vi "tokenizer.vi"(1 "Input String":string) -> (0 "Output Array":string[](array[string]))   [LabVIEW 2010]
uses:
  <vilib>/Utility/error.llb/whitespace.ctl
panel:
  out "Token":string
  out "Output":string
  # "1) LINE<space>[Displacement]<space>[Speed]<space>[Current]"
  # "2) JUMP<space>[Displacement]<space>[Speed]"
  # "3) ARC<space>[Type]<space>[Radius]<space>[Current]"
  # "4) LINE1<space>[Displacement]<space>[Speed]<space>[Current]<space>[t_before]<space>[t_enable]<space>[Frequency]<space>[DTY]<space>[HIL]<space>[LOL]"
  # "5) LINE2<space>[Displacement]<space>[Speed]<space>[Current]<space>[t_before]<space>[frequency]<space>[Amplitude]<space>[t_enable]"
  # "6) WAIT<space>[Time]"
  # "1"
  # "2"
  # "3"
  # "4"
  # "5"
  # "6"
  # "7"
  # "8"
  # "9"
  # "10"
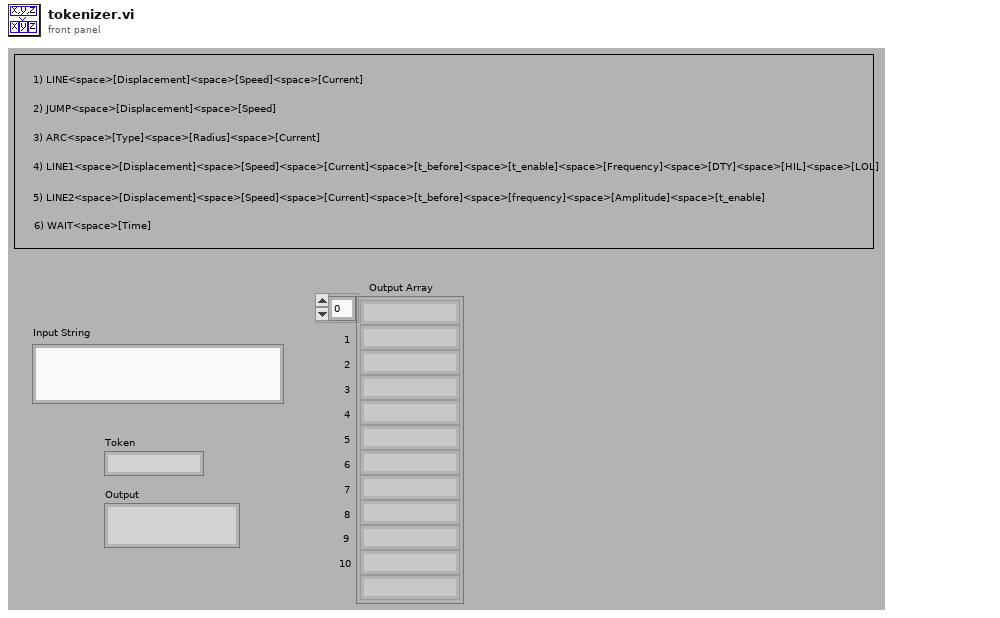
[diagram p1: front panel]
types:
  T1 = typedef "whitespace.ctl" = u16
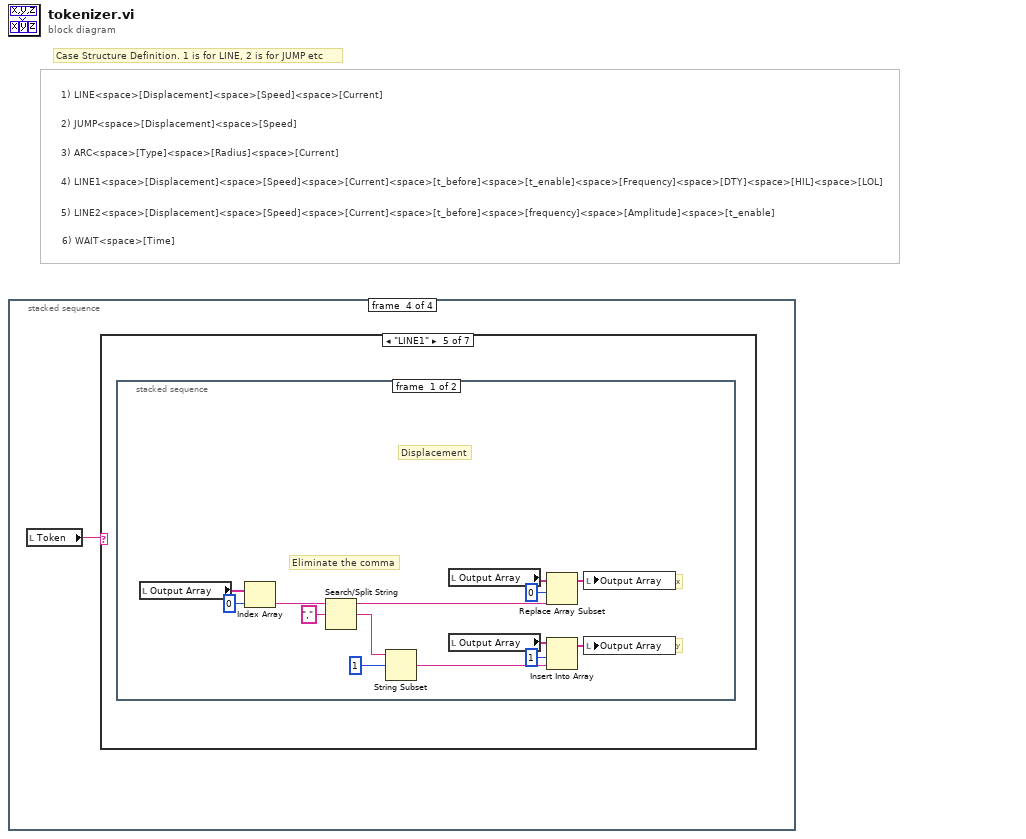
[diagram p0: block diagram]
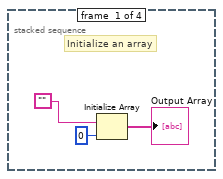
[diagram p2: hidden frame]
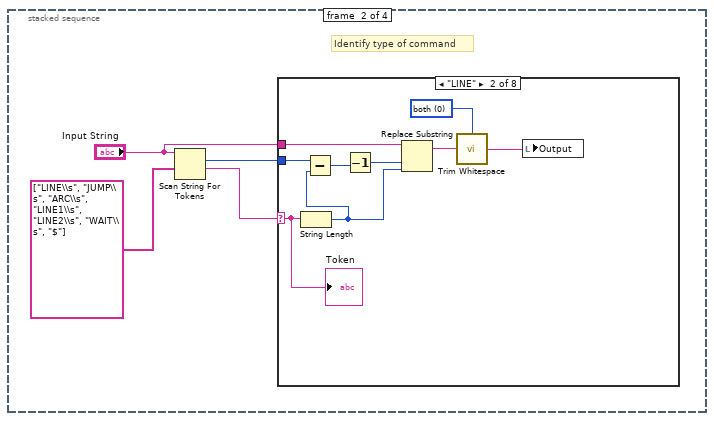
[diagram p3: hidden frame]
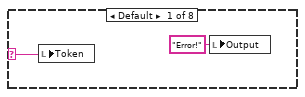
[diagram p4: hidden frame]
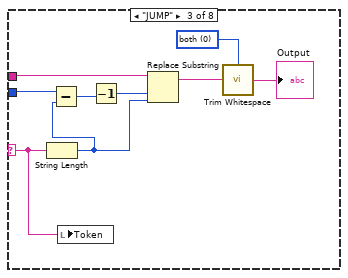
[diagram p5: hidden frame]
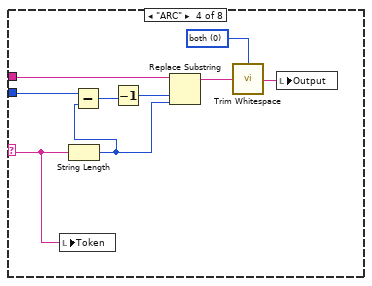
[diagram p6: hidden frame]
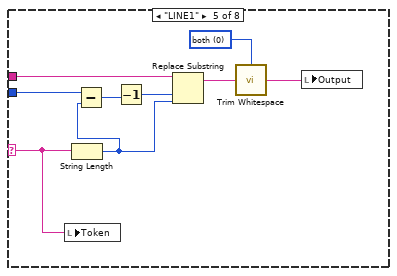
[diagram p7: hidden frame]
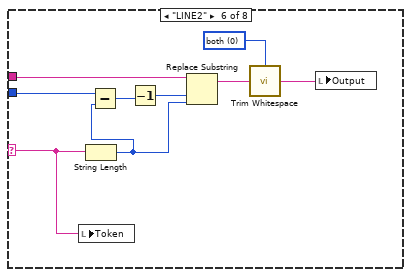
[diagram p8: hidden frame]
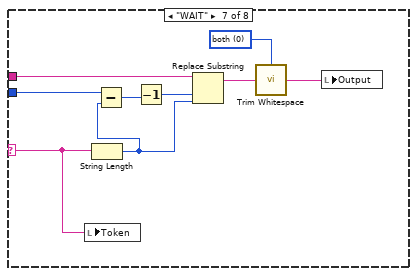
[diagram p9: hidden frame]
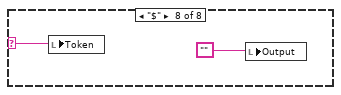
[diagram p10: hidden frame]
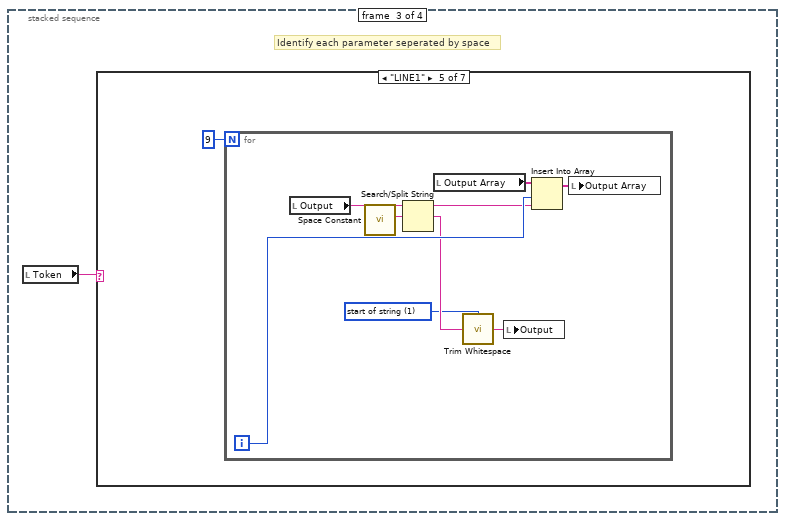
[diagram p11: hidden frame]
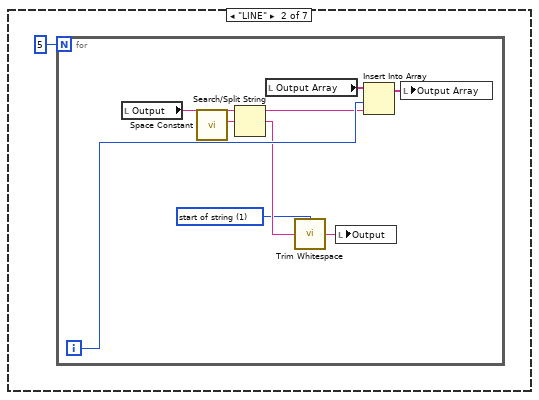
[diagram p13: hidden frame]
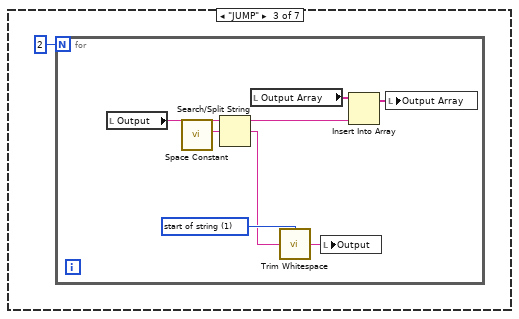
[diagram p14: hidden frame]
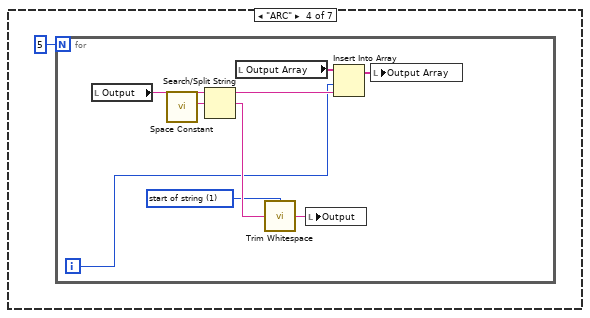
[diagram p15: hidden frame]
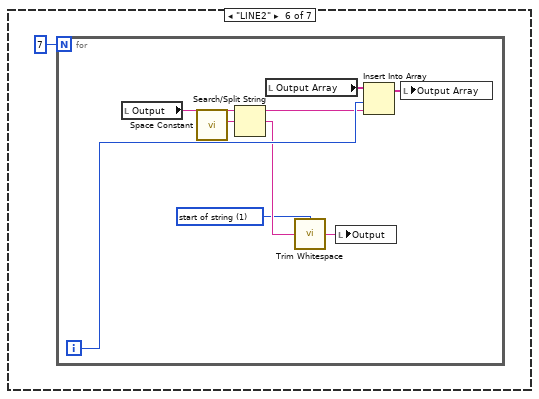
[diagram p16: hidden frame]
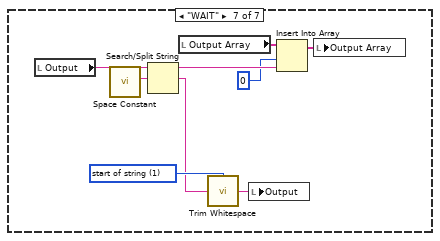
[diagram p17: hidden frame]
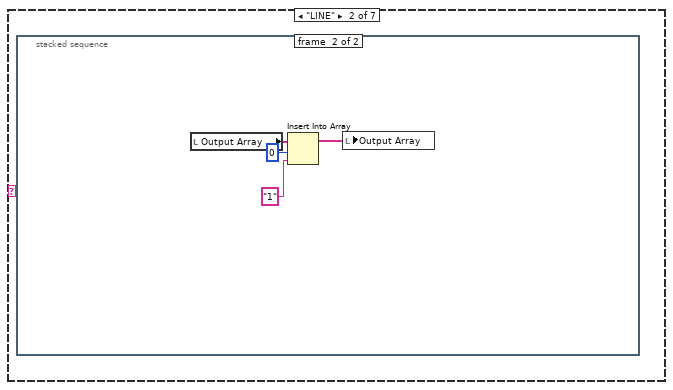
[diagram p19: hidden frame]
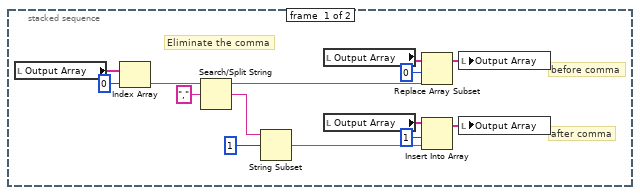
[diagram p20: hidden frame]
diagram:
  # "Case Structure Definition. 1 is for LINE, 2 is for JUMP etc"
  # "6) WAIT<space>[Time]"
  # "5) LINE2<space>[Displacement]<space>[Speed]<space>[Current]<space>[t_before]<space>[frequency]<space>[Amplitude]<space>[t_enable]"
  # "4) LINE1<space>[Displacement]<space>[Speed]<space>[Current]<space>[t_before]<space>[t_enable]<space>[Frequency]<space>[DTY]<space>[HIL]<space>[LOL]"
  # "3) ARC<space>[Type]<space>[Radius]<space>[Current]"
  # "2) JUMP<space>[Displacement]<space>[Speed]"
  # "1) LINE<space>[Displacement]<space>[Speed]<space>[Current]"
  n1 = stacked-sequence {
    frame #0 {
      # "Initialize an array"
      n2 = Initialize Array("", 0 ("dimension size")) -> (→"Output Array":string[])
    }
    frame #1 {
      # "Identify type of command"
      n3 = Scan String For Tokens(7:string[] ["LINE\\s", "JUMP\\s", "ARC\\s", "LINE1\\s", "LINE2\\s", "WAIT\\s", "$"] ("operators (none)"), 9:"Input String") -> (1:w7:string, 2:w5:i32)  [unwired: 4 in, 2 out]
      n4 = case shown="\"LINE\"" w7 {
        selector: w7 -> [w8 w13 w22 w31 w40 w47 w55 w65]
        tunnel: "Input String" -> [_ w18 w24 w33 w42 w49 w57 _]
        tunnel: w5 -> [_ w17 w23 w32 w41 w48 w56 _]
        frame Default {
          n5 = local write "Token"(w8) -> ()
          n6 = local write "Output"("Error!" ("String")) -> ()
        }
        frame "LINE" {
          w10 = T1 0 items=["both", "start of string", "end of string"] ("location (both)")
          n7 = String Length(string=w13) -> (length=w16:i32)
          n8 = Subtract(x=w17, y=w16) -> (x-y=w15:i32)
          n9 = Decrement(x=w15) -> (x-1=w14:i32)
          n10 = Replace Substring(2:w16, 3:w14, 5:w18) -> (1:w12:string)  [unwired: 1 in, 1 out]
          n11 = call <vilib>:"Trim Whitespace.vi"("string"=w12, "location (both)"=w10) -> ("trimmed string"=w11:string)
          n12 = local write "Output"(w11) -> ()
          "Token" <- w13
        }
        frame "JUMP" {
          w21 = T1 0 items=["both", "start of string", "end of string"] ("location (both)")
          n13 = String Length(string=w22) -> (length=w27:i32)
          n14 = Subtract(x=w23, y=w27) -> (x-y=w26:i32)
          n15 = local write "Token"(w22) -> ()
          n16 = Decrement(x=w26) -> (x-1=w25:i32)
          n17 = Replace Substring(2:w27, 3:w25, 5:w24) -> (1:w20:string)  [unwired: 1 in, 1 out]
          n18 = call <vilib>:"Trim Whitespace.vi"("string"=w20, "location (both)"=w21) -> ("trimmed string"=→"Output":string)
        }
        frame "ARC" {
          w30 = T1 0 items=["both", "start of string", "end of string"] ("location (both)")
          n19 = local write "Token"(w31) -> ()
          n20 = String Length(string=w31) -> (length=w36:i32)
          n21 = Subtract(x=w32, y=w36) -> (x-y=w35:i32)
          n22 = Decrement(x=w35) -> (x-1=w34:i32)
          n23 = Replace Substring(2:w36, 3:w34, 5:w33) -> (1:w28:string)  [unwired: 1 in, 1 out]
          n24 = call <vilib>:"Trim Whitespace.vi"("string"=w28, "location (both)"=w30) -> ("trimmed string"=w29:string)
          n25 = local write "Output"(w29) -> ()
        }
        frame "LINE1" {
          w38 = T1 0 items=["both", "start of string", "end of string"] ("location (both)")
          n26 = local write "Token"(w40) -> ()
          n27 = String Length(string=w40) -> (length=w45:i32)
          n28 = Subtract(x=w41, y=w45) -> (x-y=w44:i32)
          n29 = Decrement(x=w44) -> (x-1=w43:i32)
          n30 = Replace Substring(2:w45, 3:w43, 5:w42) -> (1:w37:string)  [unwired: 1 in, 1 out]
          n31 = call <vilib>:"Trim Whitespace.vi"("string"=w37, "location (both)"=w38) -> ("trimmed string"=w39:string)
          n32 = local write "Output"(w39) -> ()
        }
        frame "LINE2" {
          w46 = T1 0 items=["both", "start of string", "end of string"] ("location (both)")
          n33 = local write "Token"(w47) -> ()
          n34 = String Length(string=w47) -> (length=w54:i32)
          n35 = Subtract(x=w48, y=w54) -> (x-y=w53:i32)
          n36 = Decrement(x=w53) -> (x-1=w52:i32)
          n37 = Replace Substring(2:w54, 3:w52, 5:w49) -> (1:w50:string)  [unwired: 1 in, 1 out]
          n38 = call <vilib>:"Trim Whitespace.vi"("string"=w50, "location (both)"=w46) -> ("trimmed string"=w51:string)
          n39 = local write "Output"(w51) -> ()
        }
        frame "WAIT" {
          w58 = T1 0 items=["both", "start of string", "end of string"] ("location (both)")
          n40 = local write "Token"(w55) -> ()
          n41 = String Length(string=w55) -> (length=w63:i32)
          n42 = Subtract(x=w56, y=w63) -> (x-y=w62:i32)
          n43 = Decrement(x=w62) -> (x-1=w61:i32)
          n44 = Replace Substring(2:w63, 3:w61, 5:w57) -> (1:w59:string)  [unwired: 1 in, 1 out]
          n45 = call <vilib>:"Trim Whitespace.vi"("string"=w59, "location (both)"=w58) -> ("trimmed string"=w60:string)
          n46 = local write "Output"(w60) -> ()
        }
        frame "$" {
          n47 = local write "Token"(w65) -> ()
          n48 = local write "Output"("") -> ()
        }
      }
    }
    frame #2 {
      # "Identify each parameter seperated by space"
      n49 = local read "Token"() -> (w66:string)
      n50 = case shown="\"LINE1\"" w66 {
        frame Default {
        }
        frame "LINE" {
          n51 = for {
            N: 5 -> [_]
            i -> [w74]
            w68 = T1 1 items=["both", "start of string", "end of string"] ("location (both)")
            n52 = local read "Output"() -> (w73:string)
            n53 = call <vilib>:"Space Constant.vi"() -> ("String"=w72:string)
            n54 = Search/Split String(string=w73, search string/char (-)=w72) -> (substring before match=w71:string, match + rest of string=w70:string)  [unwired: 1 in, 1 out]
            n55 = local read "Output Array"() -> (w76:string[])
            n56 = call <vilib>:"Trim Whitespace.vi"("string"=w70, "location (both)"=w68) -> ("trimmed string"=w69:string)
            n57 = local write "Output"(w69) -> ()
            n58 = Insert Into Array(array=w76, index=w74, new element=w71) -> (w75:string[])
            n59 = local write "Output Array"(w75) -> ()
          }
        }
        frame "JUMP" {
          n60 = for {
            N: 2 -> [_]
            w85 = T1 1 items=["both", "start of string", "end of string"] ("location (both)")
            n61 = local read "Output"() -> (w80:string)
            n62 = call <vilib>:"Space Constant.vi"() -> ("String"=w81:string)
            n63 = Search/Split String(string=w80, search string/char (-)=w81) -> (substring before match=w82:string, match + rest of string=w83:string)  [unwired: 1 in, 1 out]
            n64 = local read "Output Array"() -> (w78:string[])
            n65 = call <vilib>:"Trim Whitespace.vi"("string"=w83, "location (both)"=w85) -> ("trimmed string"=w84:string)
            n66 = local write "Output"(w84) -> ()
            n67 = Insert Into Array(array=w78, new element=w82) -> (w79:string[])  [unwired: 1 in]
            n68 = local write "Output Array"(w79) -> ()
          }
        }
        frame "ARC" {
          n69 = for {
            N: 5 -> [_]
            i -> [w87]
            w88 = T1 1 items=["both", "start of string", "end of string"] ("location (both)")
            n70 = local read "Output"() -> (w93:string)
            n71 = call <vilib>:"Space Constant.vi"() -> ("String"=w92:string)
            n72 = Search/Split String(string=w93, search string/char (-)=w92) -> (substring before match=w91:string, match + rest of string=w90:string)  [unwired: 1 in, 1 out]
            n73 = local read "Output Array"() -> (w95:string[])
            n74 = call <vilib>:"Trim Whitespace.vi"("string"=w90, "location (both)"=w88) -> ("trimmed string"=w89:string)
            n75 = local write "Output"(w89) -> ()
            n76 = Insert Into Array(array=w95, index=w87, new element=w91) -> (w94:string[])
            n77 = local write "Output Array"(w94) -> ()
          }
        }
        frame "LINE1" {
          n78 = for {
            N: 9 -> [_]
            i -> [w103]
            w97 = T1 1 items=["both", "start of string", "end of string"] ("location (both)")
            n79 = local read "Output"() -> (w102:string)
            n80 = call <vilib>:"Space Constant.vi"() -> ("String"=w101:string)
            n81 = Search/Split String(string=w102, search string/char (-)=w101) -> (substring before match=w100:string, match + rest of string=w99:string)  [unwired: 1 in, 1 out]
            n82 = local read "Output Array"() -> (w105:string[])
            n83 = call <vilib>:"Trim Whitespace.vi"("string"=w99, "location (both)"=w97) -> ("trimmed string"=w98:string)
            n84 = local write "Output"(w98) -> ()
            n85 = Insert Into Array(array=w105, index=w103, new element=w100) -> (w104:string[])
            n86 = local write "Output Array"(w104) -> ()
          }
        }
        frame "LINE2" {
          n87 = for {
            N: 7 -> [_]
            i -> [w113]
            w107 = T1 1 items=["both", "start of string", "end of string"] ("location (both)")
            n88 = local read "Output"() -> (w112:string)
            n89 = call <vilib>:"Space Constant.vi"() -> ("String"=w111:string)
            n90 = Search/Split String(string=w112, search string/char (-)=w111) -> (substring before match=w110:string, match + rest of string=w109:string)  [unwired: 1 in, 1 out]
            n91 = local read "Output Array"() -> (w115:string[])
            n92 = call <vilib>:"Trim Whitespace.vi"("string"=w109, "location (both)"=w107) -> ("trimmed string"=w108:string)
            n93 = local write "Output"(w108) -> ()
            n94 = Insert Into Array(array=w115, index=w113, new element=w110) -> (w114:string[])
            n95 = local write "Output Array"(w114) -> ()
          }
        }
        frame "WAIT" {
          w124 = T1 1 items=["both", "start of string", "end of string"] ("location (both)")
          n96 = local read "Output"() -> (w119:string)
          n97 = call <vilib>:"Space Constant.vi"() -> ("String"=w120:string)
          n98 = Search/Split String(string=w119, search string/char (-)=w120) -> (substring before match=w121:string, match + rest of string=w122:string)  [unwired: 1 in, 1 out]
          n99 = local read "Output Array"() -> (w117:string[])
          n100 = call <vilib>:"Trim Whitespace.vi"("string"=w122, "location (both)"=w124) -> ("trimmed string"=w123:string)
          n101 = local write "Output"(w123) -> ()
          n102 = Insert Into Array(array=w117, index=0, new element=w121) -> (w118:string[])
          n103 = local write "Output Array"(w118) -> ()
        }
      }
    }
    frame #3 {
      n104 = local read "Token"() -> (w125:string)
      n105 = case shown="\"LINE1\"" w125 {
        frame Default {
        }
        frame "LINE" {
          n106 = stacked-sequence {
            frame #0 {
              # "after comma"
              # "before comma"
              # "Eliminate the comma"
              n107 = local read "Output Array"() -> (w138:string[])
              n108 = Index Array(array=w138, index=0) -> (element=w136:string)
              n109 = Search/Split String(string=w136, search string/char (-)=",") -> (substring before match=w132:string, match + rest of string=w130:string)  [unwired: 1 in, 1 out]
              n110 = String Subset(string=w130, offset (0)=1 ("length (rest)")) -> (substring=w129:string)  [unwired: 1 in]
              n111 = local read "Output Array"() -> (w134:string[])
              n112 = local read "Output Array"() -> (w139:string[])
              n113 = Replace Array Subset(array=w134, new element=w132, index=0) -> (w133:string[])
              n114 = Insert Into Array(array=w139, index=1, new element=w129) -> (w126:string[])
              n115 = local write "Output Array"(w133) -> ()
              n116 = local write "Output Array"(w126) -> ()
            }
            frame #1 {
              n117 = local read "Output Array"() -> (w143:string[])
              n118 = Insert Into Array(array=w143, index=0, new element="1" ("new element/subarray")) -> (w142:string[])
              n119 = local write "Output Array"(w142) -> ()
            }
          }
        }
        frame "JUMP" {
          n120 = stacked-sequence {
            frame #0 {
              # "after comma"
              # "before comma"
              # "Eliminate the comma"
              n121 = local read "Output Array"() -> (w156:string[])
              n122 = Index Array(array=w156, index=0) -> (element=w154:string)
              n123 = Search/Split String(string=w154, search string/char (-)=",") -> (substring before match=w150:string, match + rest of string=w148:string)  [unwired: 1 in, 1 out]
              n124 = String Subset(string=w148, offset (0)=1 ("length (rest)")) -> (substring=w147:string)  [unwired: 1 in]
              n125 = local read "Output Array"() -> (w152:string[])
              n126 = local read "Output Array"() -> (w157:string[])
              n127 = Replace Array Subset(array=w152, new element=w150, index=0) -> (w151:string[])
              n128 = Insert Into Array(array=w157, index=1, new element=w147) -> (w144:string[])
              n129 = local write "Output Array"(w151) -> ()
              n130 = local write "Output Array"(w144) -> ()
            }
            frame #1 {
              n131 = local read "Output Array"() -> (w161:string[])
              n132 = Insert Into Array(array=w161, index=0, new element="2" ("new element/subarray")) -> (w160:string[])
              n133 = local write "Output Array"(w160) -> ()
            }
          }
        }
        frame "ARC" {
          n134 = local read "Output Array"() -> (w165:string[])
          n135 = Insert Into Array(array=w165, index=0, new element="3" ("new element/subarray")) -> (w164:string[])
          n136 = local write "Output Array"(w164) -> ()
        }
        frame "LINE1" {
          n137 = stacked-sequence {
            frame #0 {
              # "Displacement"
              # "y"
              # "x"
              # "Eliminate the comma"
              n138 = local read "Output Array"() -> (w178:string[])
              n139 = Index Array(array=w178, index=0) -> (element=w176:string)
              n140 = Search/Split String(string=w176, search string/char (-)=",") -> (substring before match=w172:string, match + rest of string=w170:string)  [unwired: 1 in, 1 out]
              n141 = String Subset(string=w170, offset (0)=1 ("length (rest)")) -> (substring=w169:string)  [unwired: 1 in]
              n142 = local read "Output Array"() -> (w174:string[])
              n143 = local read "Output Array"() -> (w179:string[])
              n144 = Replace Array Subset(array=w174, new element=w172, index=0) -> (w173:string[])
              n145 = Insert Into Array(array=w179, index=1, new element=w169) -> (w166:string[])
              n146 = local write "Output Array"(w173) -> ()
              n147 = local write "Output Array"(w166) -> ()
            }
            frame #1 {
              n148 = local read "Output Array"() -> (w183:string[])
              n149 = Insert Into Array(array=w183, index=0, new element="4" ("new element/subarray")) -> (w182:string[])
              n150 = local write "Output Array"(w182) -> ()
            }
          }
        }
        frame "LINE2" {
          n151 = stacked-sequence {
            frame #0 {
              # "Displacement"
              # "y"
              # "x"
              # "Eliminate the comma"
              n152 = local read "Output Array"() -> (w196:string[])
              n153 = Index Array(array=w196, index=0) -> (element=w194:string)
              n154 = Search/Split String(string=w194, search string/char (-)=",") -> (substring before match=w190:string, match + rest of string=w188:string)  [unwired: 1 in, 1 out]
              n155 = String Subset(string=w188, offset (0)=1 ("length (rest)")) -> (substring=w187:string)  [unwired: 1 in]
              n156 = local read "Output Array"() -> (w192:string[])
              n157 = local read "Output Array"() -> (w197:string[])
              n158 = Replace Array Subset(array=w192, new element=w190, index=0) -> (w191:string[])
              n159 = Insert Into Array(array=w197, index=1, new element=w187) -> (w184:string[])
              n160 = local write "Output Array"(w191) -> ()
              n161 = local write "Output Array"(w184) -> ()
            }
            frame #1 {
              n162 = local read "Output Array"() -> (w201:string[])
              n163 = Insert Into Array(array=w201, index=0, new element="5" ("new element/subarray")) -> (w200:string[])
              n164 = local write "Output Array"(w200) -> ()
            }
          }
        }
        frame "WAIT" {
          n165 = stacked-sequence {
            frame #0 {
              n166 = local read "Output Array"() -> (w205:string[])
              n167 = Insert Into Array(array=w205, index=0, new element="6" ("new element/subarray")) -> (w204:string[])
              n168 = local write "Output Array"(w204) -> ()
            }
            frame #1 {
              n169 = for {
                N: 3 -> [_]
                i -> [w209]
                n170 = local read "Output Array"() -> (w212:string[])
                n171 = Add(x=2, y=w209) -> (x+y=w207:i32)
                n172 = Insert Into Array(array=w212, index=w207, new element="") -> (w211:string[])
                n173 = local write "Output Array"(w211) -> ()
              }
            }
          }
        }
      }
    }
  }
